vi "Display Mode.vi"(8 "error in (no error)":errorcluster, 10 "Display Mode":bool, 11 "Controller in":refnum<class "Controller.lvclass">) -> (0 "error out":errorcluster, 3 "Controller out":refnum<class "Controller.lvclass">)   [LabVIEW 2022 SP3, in "Controller.lvlib" / "Controller.lvclass"]
uses:
  Controller.lvclass
  Controller.lvclass/Controller.ctl
  ImageHandler/ImageHandler Messages/Display Mode Msg/Display Mode Msg.lvclass
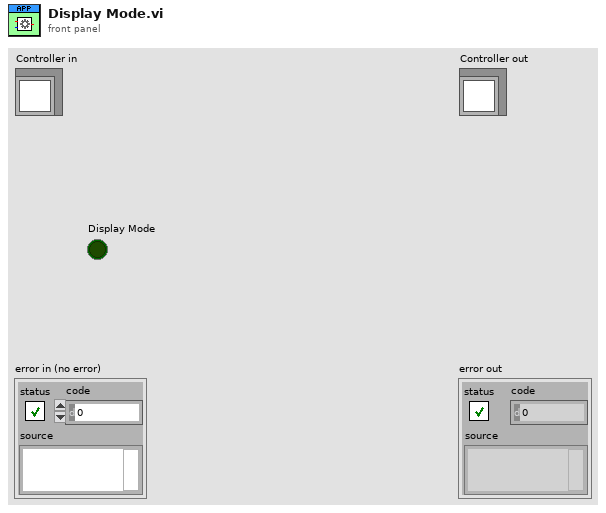
[diagram p1: front panel]
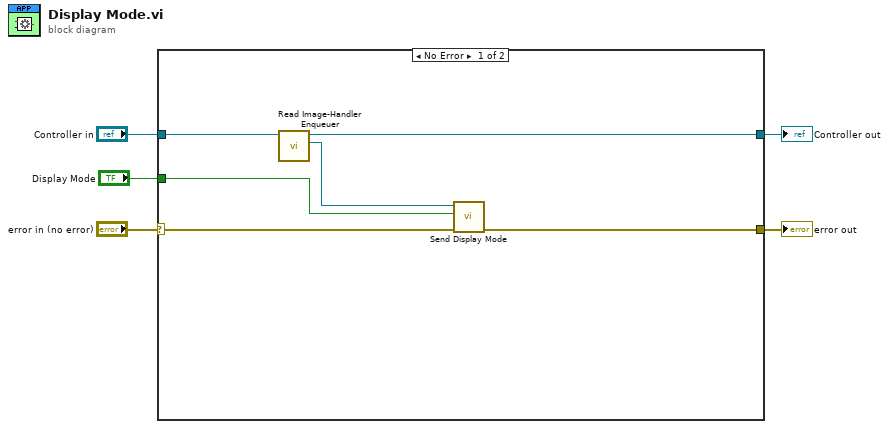
[diagram p0: block diagram]
diagram:
  n1 = case shown="No Error" "error in (no error)" {
    selector: "error in (no error)" -> [w7 w12]
    tunnel: "Controller in" -> [w11 w13]
    tunnel: [w10 w13] -> w4
    tunnel: [w6 w12] -> w2
    tunnel: "Display Mode" -> [w8 _]
    frame No Error {
      n2 = call "Read Image-Handler Enqueuer.vi"("Controller in"=w11) -> ("Actor Framework:Message Enqueuer"=w9:refnum<class "Message Enqueuer.lvclass">, "Controller out"=w10:refnum<class "Controller.lvclass">)  [unwired: 8 in, 1 out]
      n3 = call "Send Display Mode.vi"("error in (no error)"=w7, "Display Mode"=w8, "Message Enqueuer"=w9) -> ("error out"=w6:errorcluster)  [unwired: 7 in, 1 out]
    }
    frame Error {
    }
  }
  "error out" <- w2
  "Controller out" <- w4
